vi "Tosca-TTL Thread.vi"(0 "TTLDevice":refnum<class "TTLControlledDevice.lvclass">, 7 "Control Queue":refnum<queue>, 11 "Thread Notifier":refnum<notifier>) -> ()   [LabVIEW 2020]
uses:
  Device Classes/Base Class/TTLControlledDevice.lvclass
  D:/Development/epl-vi-lib/Koop/KObject Class/KObject.lvclass
  Control Classes/Base Class/TTLController.lvclass
  Device Classes/Base Class/TTLControlledDevice.lvclass/TTLControlledDevice.ctl
  Control Classes/Base Class/TTLController.lvclass/TTLController.ctl
  Trace VIs/Tosca-Trace-Event.ctl
  Control Classes/TCPController/TCPController.lvclass
  D:/Development/epl-tosca/LV Source/TTL VIs/Control Classes/Base Class/TTLController.lvclass
  Control Classes/TCPController/TCPController.lvclass/TCPController.ctl
  <vilib>/DAQmx/write.llb/DAQmx Write (Digital Bool 1Line 1Point).vi
  Control Classes/Base Class/Read When.vi
  Control Classes/Base Class/Read StartVal.vi
  Control Classes/Base Class/Read Start When.vi
  Control Classes/Base Class/Read StopVal.vi
  Control Classes/Base Class/Read Active.vi
  Control Classes/Base Class/Read Pulse.vi
  Control Classes/Base Class/Read Name.vi
  Device Classes/Base Class/Read Line.vi
  Control Classes/TCPController/Read TCPStart.vi
  <vilib>/DAQmx/create/channels.llb/DAQmx Create Channel (DO-Digital Output).vi
  <vilib>/DAQmx/miscellaneous.llb/DAQmx Fill In Error Info.vi
  epl-vi-lib/Utility VIs/User Variables/UserVars-Expression to Vector (V2).vi
  epl-vi-lib/Utility VIs/Array Manipulation VIs/Array-Last Value.vi
  epl-vi-lib/Koop/KObject Class/KObject.lvclass
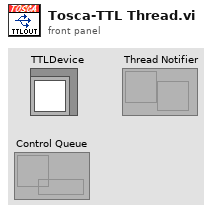
[diagram p1: front panel]
types:
  T1 = typedef "Tosca-Trace-Event.ctl" = enum16{"Unspecified", "Trial start", "Enqueue", "Result", "End parser", "Frame", "Queue available", "Timeout sent", "WritePos", "TTL"}
  T2 = enum16{"big-endian, network order", "native, host order", "little-endian"}
  T3 = typedef "TTLController.lvclass/Pulse.ctl" = cluster{"Active":bool, "IPI":string, "Width (ms)":dbl}
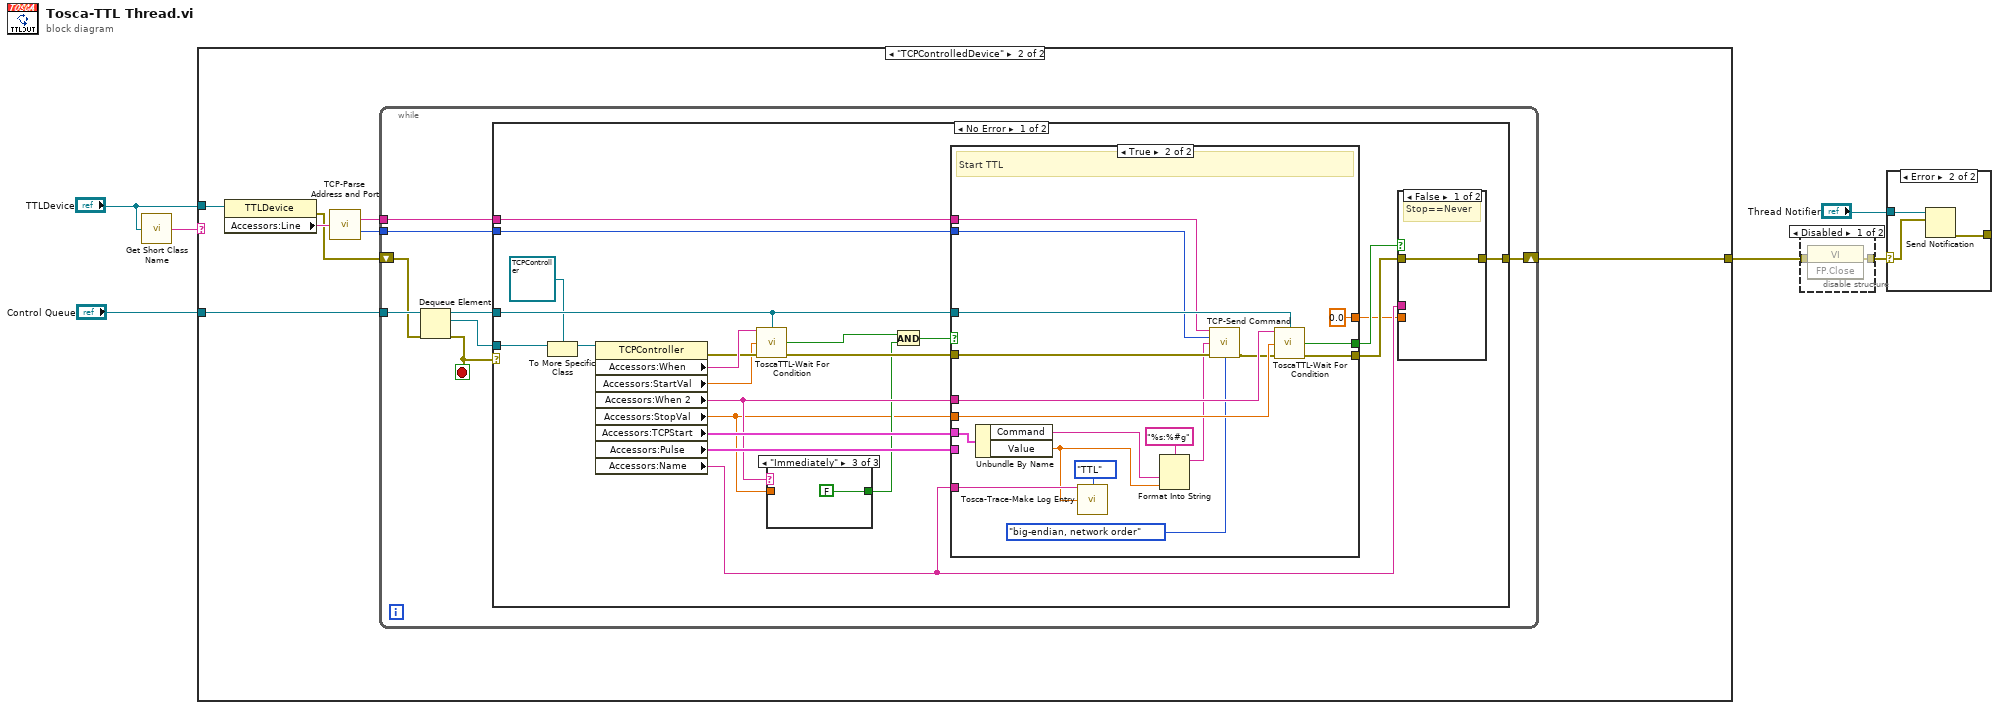
[diagram p0: block diagram]
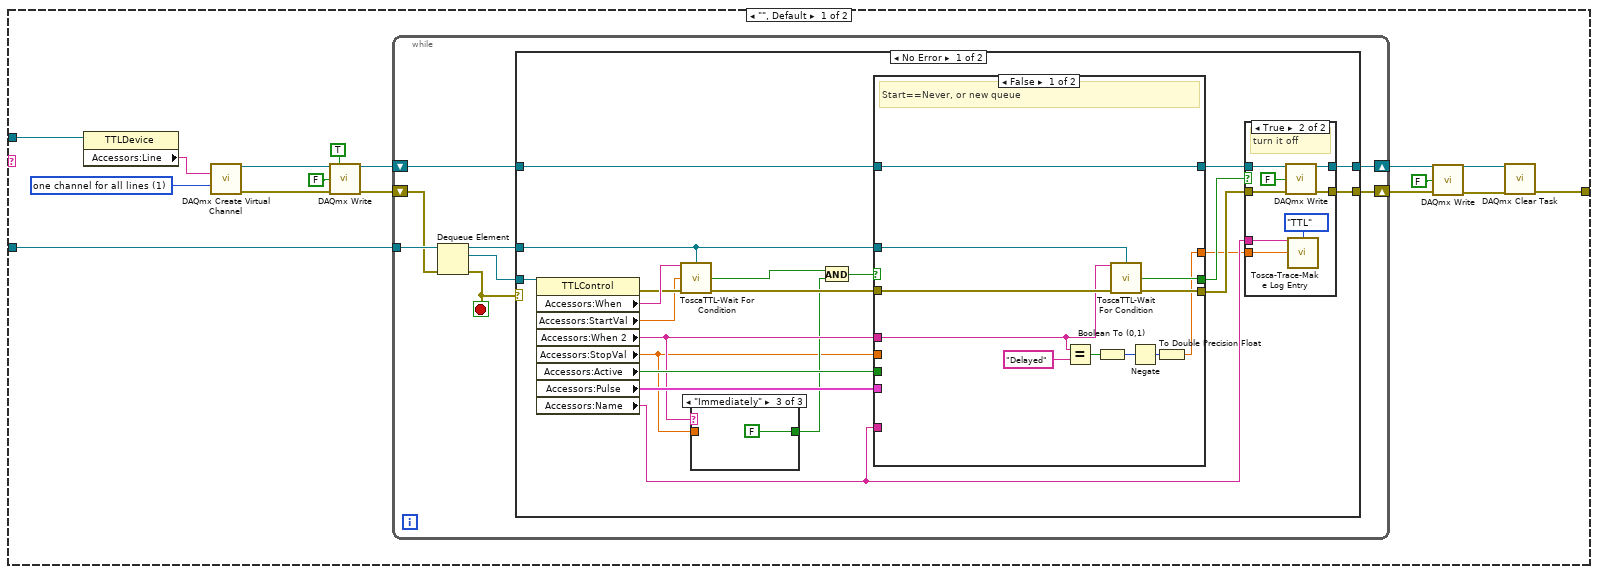
[diagram p2: hidden frame]
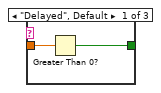
[diagram p3: hidden frame]
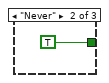
[diagram p4: hidden frame]
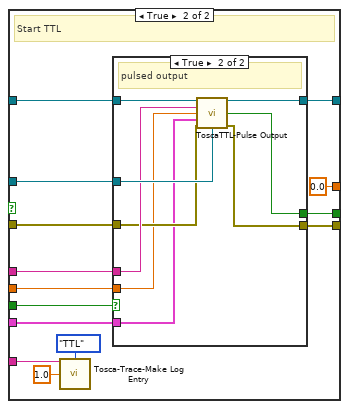
[diagram p5: hidden frame]
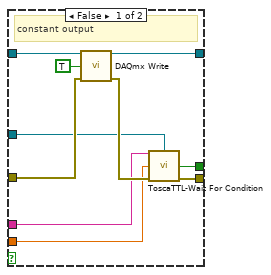
[diagram p6: hidden frame]
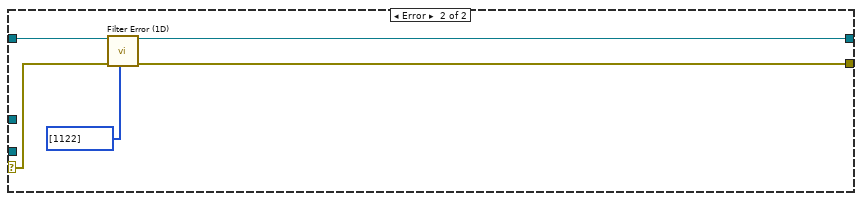
[diagram p8: hidden frame]
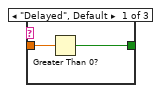
[diagram p9: hidden frame]
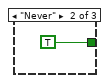
[diagram p10: hidden frame]
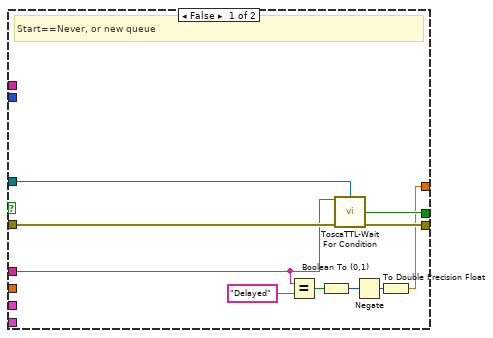
[diagram p11: hidden frame]
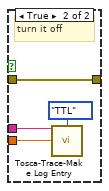
[diagram p12: hidden frame]
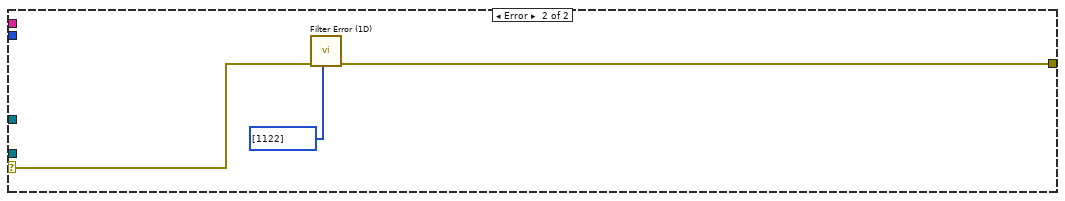
[diagram p13: hidden frame]
diagram:
  n1 = call "Get Short Class Name.vi"("KObject in"="TTLDevice") -> ("Class"=w1:string)  [unwired: 4 in]
  n2 = case shown="\"TCPControlledDevice\"" w1 {
    tunnel: "TTLDevice" -> [w16 w120]
    tunnel: [w8 w114] -> w6
    tunnel: "Control Queue" -> [w7 w119]
    frame "", Default {
      w19 = 1 items=["one channel for each line", "one channel for all lines"] ("line grouping")
      n3 = property class="TTLDevice"(reference=w16) -> ("Accessors:Line"=w18:string)  [unwired: 1 in, 2 out]
      n4 = call-poly <vilib>:"DAQmx Create Virtual Channel.vi"("lines"=w18, "line grouping"=w19) -> ("task out"=w20:refnum<k21>, "error out"=w21:errorcluster)  [unwired: 12 in]
      n5 = call-poly <vilib>:"DAQmx Write.vi"("task/channels in"=w20, "auto start"=TRUE, "data"=FALSE, "error in"=w21) -> ("task out"=w14:refnum<k21>, "error out"=w15:errorcluster)  [unwired: 9 in, 1 out]
      n6 = while {
        tunnel: w7 -> [w30]
        shift-right: [w24] -> w12
        shift-left: w15 -> [w27]
        shift-right: [w25] -> w9
        shift-left: w14 -> [w26]
        stop <- w29 stop-if-true
        n7 = Dequeue Element(queue=w30, error in (no error)=w27) -> (queue out=w23:refnum<queue>, element=w28:refnum<class "TTLController.lvclass">, error out=w29:errorcluster)  [unwired: 1 in, 1 out]
        n8 = case shown="No Error" w29 {
          selector: w29 -> [_ w112]
          tunnel: w28 -> [w51 _]
          tunnel: w26 -> [w49 w113]
          tunnel: [w46 w113] -> w25
          tunnel: [w44 w111] -> w24
          tunnel: w23 -> [w40 _]
          frame No Error {
            n9 = property class="TTLControl"(reference=w51) -> (error out=w42:errorcluster, "Accessors:When"=w50:string, "Accessors:StartVal"=w38:dbl, "Accessors:When 2"=w37:string, "Accessors:StopVal"=w35:dbl, "Accessors:Active"=w41:bool, "Accessors:Pulse"=w39:T3, "Accessors:Name"=w32:string)  [unwired: 1 in, 1 out]
            n10 = call "ToscaTTL-Wait For Condition.vi"("When"=w50, "Control Queue"=w40, "Value"=w38, "error in (no error)"=w42) -> ("trigger"=w43:bool, "error out"=w48:errorcluster)  [unwired: 10 in]
            n11 = case shown="\"Immediately\"" w37 {
              tunnel: [w52 TRUE FALSE] -> w36
              tunnel: w35 -> [w53 _ _]
              frame "Delayed", Default {
                n12 = Greater Than 0?(x=w53) -> (x > 0?=w52:bool)
              }
              frame "Never" {
              }
              frame "Immediately" {
              }
            }
            n13 = And(x=w43, y=w36) -> (x .and. y?=w33:bool)
            n14 = case shown="False" w33 {
              tunnel: w49 -> [w66 w80]
              tunnel: w48 -> [w65 w70]
              tunnel: w37 -> [w61 w79]
              tunnel: [w66 w78] -> w47
              tunnel: [w63 w77] -> w45
              tunnel: [w64 w76] -> w34
              tunnel: w41 -> [_ w75]
              tunnel: w40 -> [w62 w74]
              tunnel: w39 -> [_ w73]
              tunnel: w35 -> [_ w72]
              tunnel: w32 -> [_ w68]
              tunnel: [w56 0.0 ("Value")] -> w31
              frame False {
                # "Start==Never, or new queue"
                n15 = Equal?(x=w61, y="Delayed") -> (x = y?=w59:bool)
                n16 = Boolean To (0,1)(Boolean=w59) -> (0, 1=w58:i16)
                n17 = call "ToscaTTL-Wait For Condition.vi"("When"=w61, "Control Queue"=w62, "error in (no error)"=w65) -> ("trigger"=w64:bool, "error out"=w63:errorcluster)  [unwired: 11 in]
                n18 = Negate(x=w58) -> (-x=w57:i16)
                n19 = To Double Precision Float(number=w57) -> (double precision float=w56:dbl)
              }
              frame True {
                # "Start TTL"
                n20 = call "Tosca-Trace-Make Log Entry.vi"("Message"=w68, "Event"=Tosca-Trace-Event."TTL", "Value"=1.0) -> ()  [unwired: 12 in, 1 out]
                n21 = case shown="True" w75 {
                  tunnel: w80 -> [w90 w99]
                  tunnel: w70 -> [w89 w94]
                  tunnel: w79 -> [w87 w96]
                  tunnel: [w86 w98] -> w78
                  tunnel: [w85 w95] -> w77
                  tunnel: [w84 w93] -> w76
                  tunnel: w74 -> [w82 w97]
                  tunnel: w73 -> [_ w91]
                  tunnel: w72 -> [w81 w92]
                  frame False {
                    # "constant output"
                    n22 = call-poly <vilib>:"DAQmx Write.vi"("task/channels in"=w90, "data"=TRUE, "error in"=w89) -> ("task out"=w86:refnum<k21>, "error out"=w88:errorcluster)  [unwired: 10 in, 1 out]
                    n23 = call "ToscaTTL-Wait For Condition.vi"("When"=w87, "Control Queue"=w82, "Value"=w81, "error in (no error)"=w88) -> ("trigger"=w84:bool, "error out"=w85:errorcluster)  [unwired: 10 in]
                  }
                  frame True {
                    # "pulsed output"
                    n24 = call "ToscaTTL-Pulse Output.vi"("task in"=w99, "StopWhen"=w96, "StopValue"=w92, "Pulse"=w91, "error in (no error)"=w94, "TTL Queue"=w97) -> ("task out"=w98:refnum<k21>, "trigger"=w93:bool, "error out"=w95:errorcluster)  [unwired: 7 in]
                  }
                }
              }
            }
            n25 = case shown="True" w34 {
              tunnel: w47 -> [w101 w109]
              tunnel: [w101 w108] -> w46
              tunnel: w45 -> [w100 w107]
              tunnel: [w100 w106] -> w44
              tunnel: w32 -> [_ w103]
              tunnel: w31 -> [_ w102]
              frame False {
                # "Stop==Never"
              }
              frame True {
                # "turn it off"
                n26 = call-poly <vilib>:"DAQmx Write.vi"("task/channels in"=w109, "data"=FALSE, "error in"=w107) -> ("task out"=w108:refnum<k21>, "error out"=w106:errorcluster)  [unwired: 10 in, 1 out]
                n27 = call "Tosca-Trace-Make Log Entry.vi"("Message"=w103, "Event"=Tosca-Trace-Event."TTL", "Value"=w102) -> ()  [unwired: 12 in, 1 out]
              }
            }
          }
          frame Error {
            n28 = call "Filter Error (1D).vi"("error in (no error)"=w112, "Array"=i32[] [1122]) -> ("error out"=w111:errorcluster)  [unwired: 9 in]
          }
        }
      }
      n29 = call-poly <vilib>:"DAQmx Write.vi"("task/channels in"=w9, "data"=FALSE, "error in"=w12) -> ("task out"=w10:refnum<k21>, "error out"=w11:errorcluster)  [unwired: 10 in, 1 out]
      n30 = call <vilib>:"DAQmx Clear Task.vi"("task in"=w10, "error in"=w11) -> ("error out"=w8:errorcluster)  [unwired: 13 in]
    }
    frame "TCPControlledDevice" {
      n31 = property class="TTLDevice"(reference=w120) -> (error out=w117:errorcluster, "Accessors:Line"=w118:string)  [unwired: 1 in, 1 out]
      n32 = call "TCP-Parse Address and Port.vi"("Address in"=w118) -> ("Address"=w116:string, "Port"=w115:i32)  [unwired: 12 in, 1 out]
      n33 = while {
        tunnel: w119 -> [w128]
        shift-right: [w124] -> w114
        shift-left: w117 -> [w125]
        tunnel: w116 -> [w122]
        tunnel: w115 -> [w121]
        stop <- w127 stop-if-true
        n34 = Dequeue Element(queue=w128, error in (no error)=w125) -> (queue out=w123:refnum<queue>, element=w126:refnum<class "TTLController.lvclass">, error out=w127:errorcluster)  [unwired: 1 in, 1 out]
        n35 = case shown="No Error" w127 {
          selector: w127 -> [_ w190]
          tunnel: w126 -> [w133 _]
          tunnel: [w147 w189] -> w124
          tunnel: w123 -> [w143 _]
          tunnel: w122 -> [w130 _]
          tunnel: w121 -> [w129 _]
          frame No Error {
            n36 = To More Specific Class(target class=refnum<class "TCPController.lvclass"> refnum ("TCPController"), reference=w133) -> (specific class reference=w131:refnum<class "TCPController.lvclass">)  [unwired: 1 in, 1 out]
            n37 = property class="TCPController"(reference=w131) -> (error out=w145:errorcluster, "Accessors:When"=w150:string, "Accessors:StartVal"=w141:dbl, "Accessors:When 2"=w140:string, "Accessors:StopVal"=w138:dbl, "Accessors:TCPStart"=w144:cluster{"Command":string, "Value":dbl}, "Accessors:Pulse"=w142:T3, "Accessors:Name"=w135:string)  [unwired: 1 in, 1 out]
            n38 = call "ToscaTTL-Wait For Condition.vi"("When"=w150, "Control Queue"=w143, "Value"=w141, "error in (no error)"=w145) -> ("trigger"=w146:bool, "error out"=w149:errorcluster)  [unwired: 10 in]
            n39 = case shown="\"Immediately\"" w140 {
              tunnel: [w151 TRUE FALSE] -> w139
              tunnel: w138 -> [w152 _ _]
              frame "Delayed", Default {
                n40 = Greater Than 0?(x=w152) -> (x > 0?=w151:bool)
              }
              frame "Never" {
              }
              frame "Immediately" {
              }
            }
            n41 = And(x=w146, y=w139) -> (x .and. y?=w136:bool)
            n42 = case shown="True" w136 {
              tunnel: w149 -> [w164 w173]
              tunnel: w140 -> [w160 w182]
              tunnel: [w162 w181] -> w148
              tunnel: [w163 w180] -> w137
              tunnel: w144 -> [_ w170]
              tunnel: w143 -> [w161 w179]
              tunnel: w142 -> [_ _]
              tunnel: w138 -> [_ w178]
              tunnel: w135 -> [_ w176]
              tunnel: [w155 0.0 ("Value")] -> w134
              tunnel: w130 -> [_ w174]
              tunnel: w129 -> [_ w171]
              frame False {
                # "Start==Never, or new queue"
                n43 = Equal?(x=w160, y="Delayed") -> (x = y?=w158:bool)
                n44 = Boolean To (0,1)(Boolean=w158) -> (0, 1=w157:i16)
                n45 = call "ToscaTTL-Wait For Condition.vi"("When"=w160, "Control Queue"=w161, "error in (no error)"=w164) -> ("trigger"=w163:bool, "error out"=w162:errorcluster)  [unwired: 11 in]
                n46 = Negate(x=w157) -> (-x=w156:i16)
                n47 = To Double Precision Float(number=w156) -> (double precision float=w155:dbl)
              }
              frame True {
                # "Start TTL"
                n48 = Unbundle By Name(w170) -> ("Command"=w168:string, "Value"=w167:dbl)
                n49 = call "Tosca-Trace-Make Log Entry.vi"("Message"=w176, "Event"=Tosca-Trace-Event."TTL", "Value"=w167) -> ()  [unwired: 12 in, 1 out]
                n50 = Format Into String(format string="%s:%#g", w168, w167) -> (resulting string=w166:string)  [unwired: 2 in, 1 out]
                n51 = call "TCP-Send Command.vi"("PXI Address"=w174, "Port"=w171, "Command"=w166, "error in (no error)"=w173, "byte order"=T2."big-endian, network order") -> ("error out"=w172:errorcluster)  [unwired: 10 in]
                n52 = call "ToscaTTL-Wait For Condition.vi"("When"=w182, "Control Queue"=w179, "Value"=w178, "error in (no error)"=w172) -> ("trigger"=w180:bool, "error out"=w181:errorcluster)  [unwired: 10 in]
              }
            }
            n53 = case shown="False" w137 {
              tunnel: w148 -> [w183 w184]
              tunnel: [w183 w184] -> w147
              tunnel: w135 -> [_ w186]
              tunnel: w134 -> [_ w185]
              frame False {
                # "Stop==Never"
              }
              frame True {
                # "turn it off"
                n54 = call "Tosca-Trace-Make Log Entry.vi"("Message"=w186, "Event"=Tosca-Trace-Event."TTL", "Value"=w185) -> ()  [unwired: 12 in, 1 out]
              }
            }
          }
          frame Error {
            n55 = call "Filter Error (1D).vi"("error in (no error)"=w190, "Array"=i32[] [1122]) -> ("error out"=w189:errorcluster)  [unwired: 9 in]
          }
        }
      }
    }
  }
  n56 = disable-structure shown="Disabled" {
    disable-tunnel: w6 -> [w192 w193]
    disable-tunnel: [w191 w193] -> w5
    frame Disabled {
      n57 = invoke class="VI" method="FP.Close"(error in=w192) -> (error out=w191:errorcluster)  [unwired: 2 in, 2 out]
    }
    frame Enabled {
    }
  }
  n58 = case shown="Error" w5 {
    selector: w5 -> [_ w195]
    tunnel: "Thread Notifier" -> [_ w196]
    tunnel: [_ w194] -> _
    frame No Error {
    }
    frame Error {
      n59 = Send Notification(notification=w195, notifier=w196) -> (error out=w194:errorcluster)  [unwired: 1 in, 1 out]
    }
  }
